vi "Convert Rectangle Data to Segment Array v2.vi"(8 "Error In":errorcluster, 9 "Box Profile Type":T1, 11 "(Rotated) Rectangle Data":i32[](array[numeric])) -> (0 "Error Out":errorcluster, 1 "Median End Points":cluster{"X":dbl, "Y":dbl}[](array[cluster]), 2 "Rectangle End Points":cluster{"X":dbl, "Y":dbl}[](array[cluster]), 3 "Rectange Profile Segments":cluster{"Segment ROI Points":i32[]}[](array[cluster]), 5 "Number of Points":i32)   [LabVIEW 2021, in "Image.lvlib"]
doc: "Converts the array of Rectangle (or Rotated Rectangle) data to an array of structures, each containing an array of (x,y) point coordinates for the corresponding \"cross-section\" segments."
uses:
  Image.lvlib
  Box Profile Type.ctl
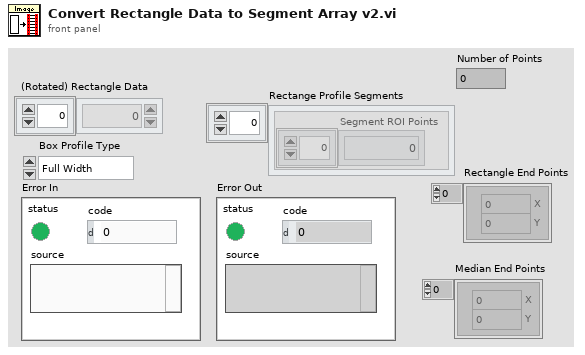
[diagram p1: front panel]
types:
  T1 = typedef "Image.lvlib/Box Profile Type.ctl" = enum16{"Full Width", "Half Width"}
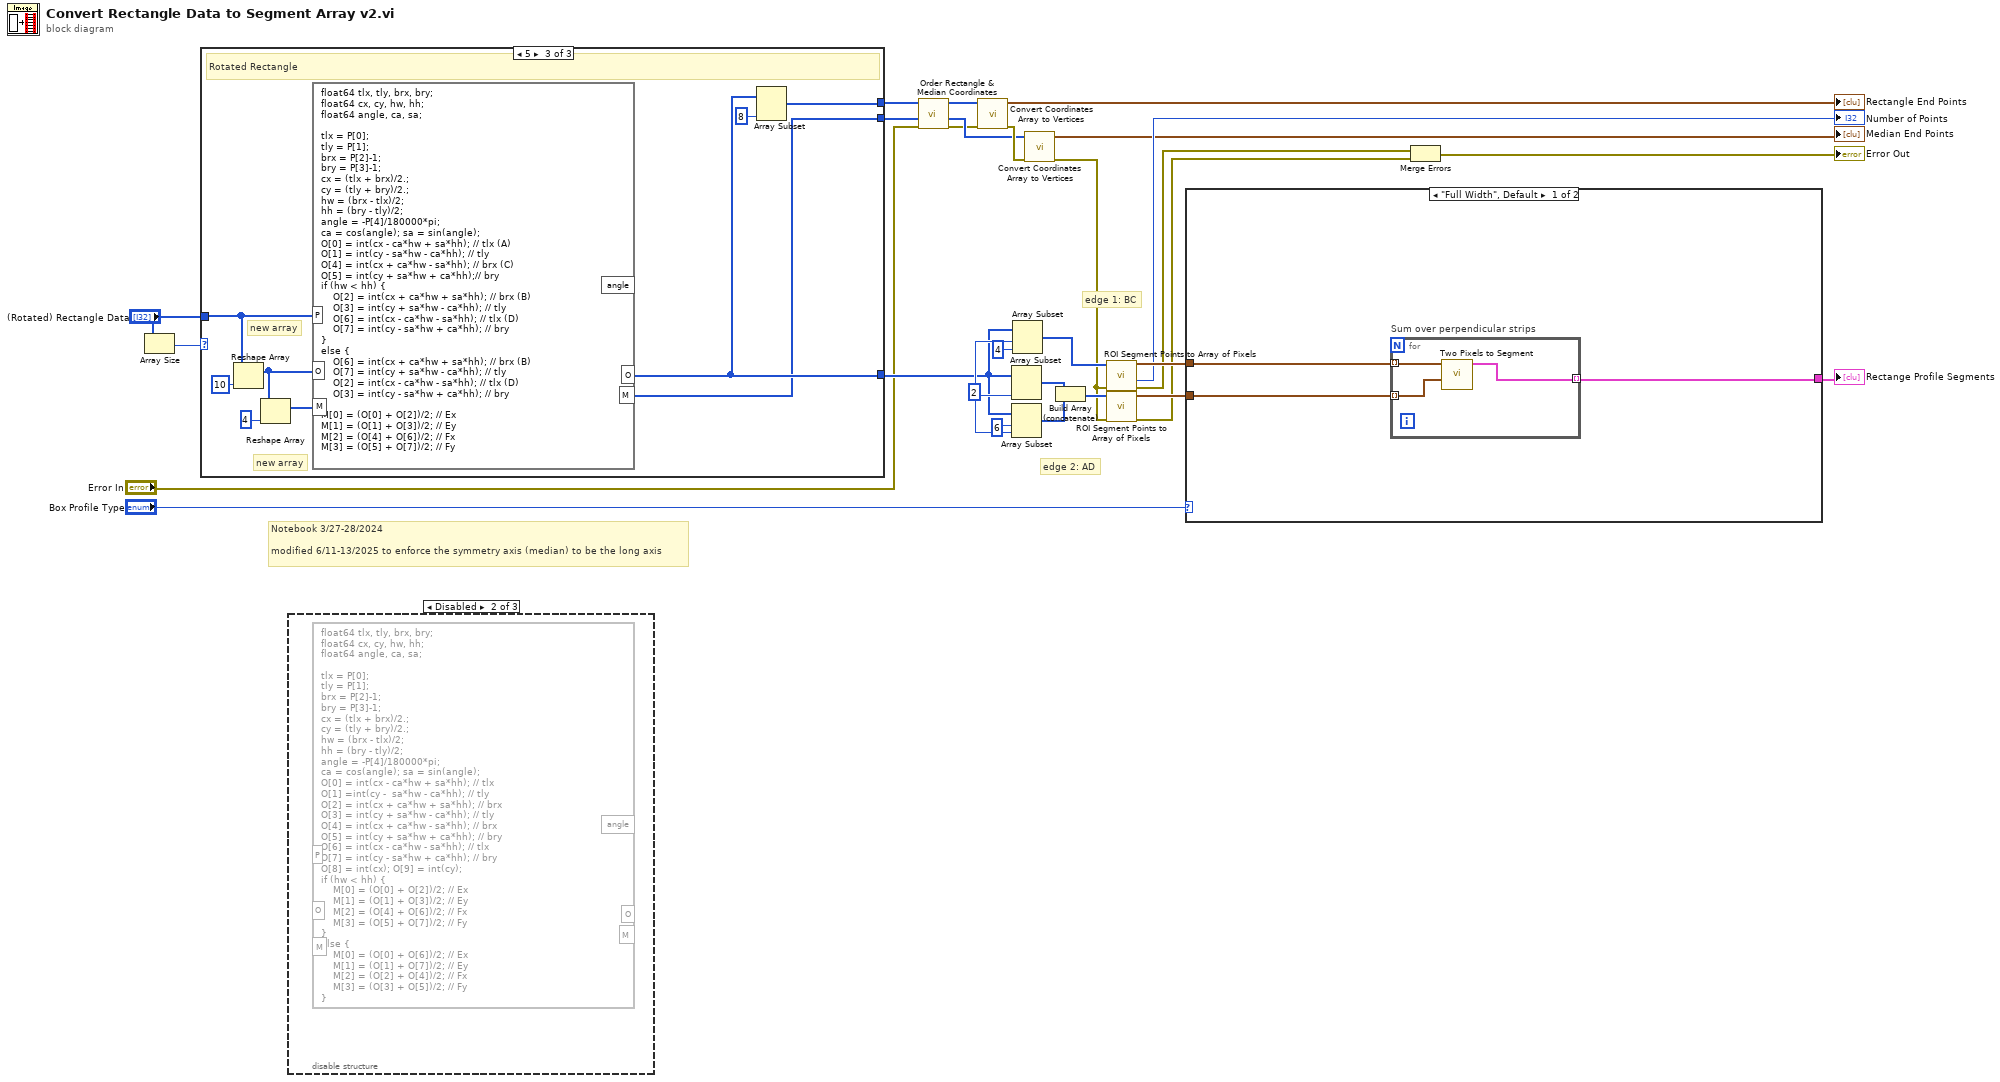
[diagram p0: block diagram]
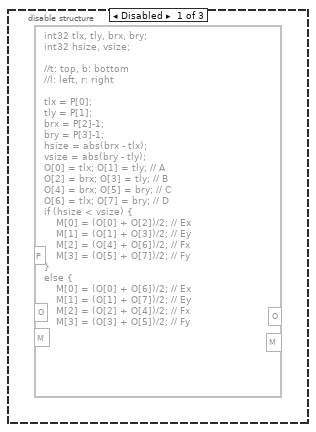
[diagram p2: hidden frame]
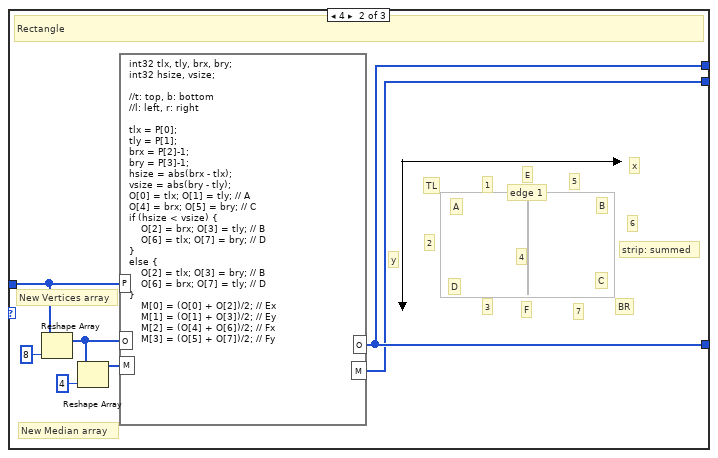
[diagram p5: hidden frame]
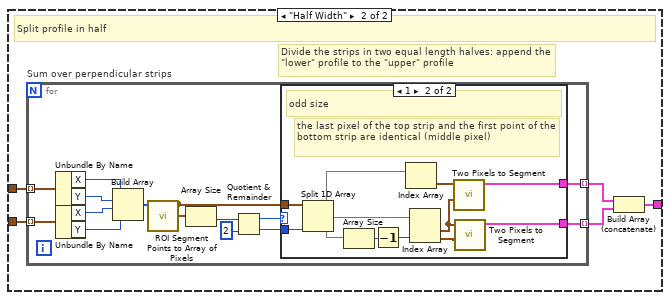
[diagram p6: hidden frame]
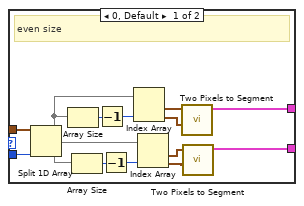
[diagram p7: hidden frame]
diagram:
  w22 = 2 ("length")
  # "edge 2: AD"
  # "edge 1: BC"
  # "Notebook 3/27-28/2024\n\nmodified 6/11-13/2025 to enforce the symmetry axis (median) to be the long axis"
  n1 = Array Size(array="(Rotated) Rectangle Data") -> (size(s)=w27:i32)
  n2 = case shown="5" w27 {
    tunnel: "(Rotated) Rectangle Data" -> [_ w35 w44]
    tunnel: [_ w33 w42] -> w12
    tunnel: [_ w33 w40] -> w6
    tunnel: [_ w29 w36] -> w5
    frame 0, Default {
    }
    frame 4 {
      # "New Median array"
      # "New Vertices array"
      # "7"
      # "6"
      # "5"
      # "4"
      # "3"
      # "2"
      # "1"
      # "F"
      # "E"
      # "strip: summed"
      # "D"
      # "C"
      # "B"
      # "A"
      # "edge 1"
      # "x"
      # "y"
      # "BR"
      # "TL"
      # "Rectangle"
      n3 = Reshape Array(w35, 8 ("dimension size")) -> (w32:i32[])
      n4 = Reshape Array(w32, 4 ("dimension size")) -> (w30:i32[])
      n5 = formula code="int32 tlx, tly, brx, bry;\nint32 hsize, vsize;\n\n//t: top, b: bottom\n//l: left, r: right\n\ntlx = P[0];\ntly = P[1];\nbrx = P[2]-1;\nbry = P[3]-1;\nhsize = abs(brx - tlx);\nvsize = abs(bry - tly);\nO[0] = tlx; O[1] = tly; // A\nO[4] = brx; O[5] = bry; // C\nif (hsize < vsize) {\n    O[2] = brx; O[3] = tly; // B\n    O[6] = tlx; O[7] = bry; // D\n}\nelse {\n    O[2] = tlx; O[3] = bry; // B\n    O[6] = brx; O[7] = tly; // D\n}\n    M[0] = (O[0] + O[2])/2; // Ex\n    M[1] = (O[1] + O[3])/2; // Ey\n    M[2] = (O[4] + O[6])/2; // Fx\n    M[3] = (O[5] + O[7])/2; // Fy"("P"=w35, "O"=w32, "M"=w30) -> ("O"=w33:i32[], "M"=w29:i32[])
    }
    frame 5 {
      # "new array"
      # "new array"
      # "Rotated Rectangle"
      n6 = Reshape Array(w44, 10 ("dimension size")) -> (w39:i32[])
      n7 = Reshape Array(w39, 4 ("dimension size")) -> (w37:i32[])
      n8 = formula code="float64 tlx, tly, brx, bry;\nfloat64 cx, cy, hw, hh;\nfloat64 angle, ca, sa;\n\ntlx = P[0];\ntly = P[1];\nbrx = P[2]-1;\nbry = P[3]-1;\ncx = (tlx + brx)/2.;\ncy = (tly + bry)/2.;\nhw = (brx - tlx)/2;\nhh = (bry - tly)/2;\nangle = -P[4]/180000*pi;\nca = cos(angle); sa = sin(angle);\nO[0] = int(cx - ca*hw + sa*hh); // tlx (A)\nO[1] = int(cy - sa*hw - ca*hh); // tly\nO[4] = int(cx + ca*hw - sa*hh); // brx (C)\nO[5] = int(cy + sa*hw + ca*hh);// bry\nif (hw < hh) {\n    O[2] = int(cx + ca*hw + sa*hh); // brx (B)\n    O[3] = int(cy + sa*hw - ca*hh); // tly\n    O[6] = int(cx - ca*hw - sa*hh); // tlx (D)\n    O[7] = int(cy - sa*hw + ca*hh); // bry\n}\nelse {\n    O[6] = int(cx + ca*hw + sa*hh); // brx (B)\n    O[7] = int(cy + sa*hw - ca*hh); // tly\n    O[2] = int(cx - ca*hw - sa*hh); // tlx (D)\n    O[3] = int(cy - sa*hw + ca*hh); // bry\n}\nM[0] = (O[0] + O[2])/2; // Ex\nM[1] = (O[1] + O[3])/2; // Ey\nM[2] = (O[4] + O[6])/2; // Fx\nM[3] = (O[5] + O[7])/2; // Fy"("P"=w44, "O"=w39, "M"=w37) -> ("O"=w42:i32[], "M"=w36:i32[])  [unwired: 1 out]
      n9 = Array Subset(array=w42, length=8) -> (w40:i32[])  [unwired: 1 in]
    }
  }
  n10 = disable-structure shown="Disabled" {
    frame Disabled {
      n11 = formula code="int32 tlx, tly, brx, bry;\nint32 hsize, vsize;\n\n//t: top, b: bottom\n//l: left, r: right\n\ntlx = P[0];\ntly = P[1];\nbrx = P[2]-1;\nbry = P[3]-1;\nhsize = abs(brx - tlx);\nvsize = abs(bry - tly);\nO[0] = tlx; O[1] = tly; // A\nO[2] = brx; O[3] = tly; // B\nO[4] = brx; O[5] = bry; // C\nO[6] = tlx; O[7] = bry; // D\nif (hsize < vsize) {\n    M[0] = (O[0] + O[2])/2; // Ex\n    M[1] = (O[1] + O[3])/2; // Ey\n    M[2] = (O[4] + O[6])/2; // Fx\n    M[3] = (O[5] + O[7])/2; // Fy\n}\nelse {\n    M[0] = (O[0] + O[6])/2; // Ex\n    M[1] = (O[1] + O[7])/2; // Ey\n    M[2] = (O[2] + O[4])/2; // Fx\n    M[3] = (O[3] + O[5])/2; // Fy\n}"() -> ()  [unwired: 3 in, 2 out]
    }
    frame Disabled {
      n12 = formula code="float64 tlx, tly, brx, bry;\nfloat64 cx, cy, hw, hh;\nfloat64 angle, ca, sa;\n\ntlx = P[0];\ntly = P[1];\nbrx = P[2]-1;\nbry = P[3]-1;\ncx = (tlx + brx)/2.;\ncy = (tly + bry)/2.;\nhw = (brx - tlx)/2;\nhh = (bry - tly)/2;\nangle = -P[4]/180000*pi;\nca = cos(angle); sa = sin(angle);\nO[0] = int(cx - ca*hw + sa*hh); // tlx\nO[1] =int(cy -  sa*hw - ca*hh); // tly\nO[2] = int(cx + ca*hw + sa*hh); // brx\nO[3] = int(cy + sa*hw - ca*hh); // tly\nO[4] = int(cx + ca*hw - sa*hh); // brx\nO[5] = int(cy + sa*hw + ca*hh); // bry\nO[6] = int(cx - ca*hw - sa*hh); // tlx\nO[7] = int(cy - sa*hw + ca*hh); // bry\nO[8] = int(cx); O[9] = int(cy);\nif (hw < hh) {\n    M[0] = (O[0] + O[2])/2; // Ex\n    M[1] = (O[1] + O[3])/2; // Ey\n    M[2] = (O[4] + O[6])/2; // Fx\n    M[3] = (O[5] + O[7])/2; // Fy\n}\nelse {\n    M[0] = (O[0] + O[6])/2; // Ex\n    M[1] = (O[1] + O[7])/2; // Ey\n    M[2] = (O[2] + O[4])/2; // Fx\n    M[3] = (O[3] + O[5])/2; // Fy\n}"() -> ()  [unwired: 3 in, 3 out]
    }
    frame Enabled {
    }
  }
  n13 = call "Order Rectangle & Median Coordinates.vi"("Error In"="Error In", "EF"=w5, "ABCD"=w6) -> ("Error Out"=w1:errorcluster, "Median"=w3:i32[], "Rectangle"=w4:i32[])  [unwired: 6 in]
  n14 = call "Convert Coordinates Array to Vertices.vi"("Error In"=w1, "Coordinates in"=w4) -> ("Error Out"=w9:errorcluster, "Vertices out"=→"Rectangle End Points":cluster{"X":dbl, "Y":dbl}[])  [unwired: 8 in]
  n15 = Array Subset(array=w12, length=w22) -> (w25:i32[])  [unwired: 1 in]
  n16 = Array Subset(array=w12, index=6, length=w22) -> (w23:i32[])
  n17 = Array Subset(array=w12, index=w22, length=4) -> (w20:i32[])
  n18 = call "Convert Coordinates Array to Vertices.vi"("Error In"=w9, "Coordinates in"=w3) -> ("Error Out"=w8:errorcluster, "Vertices out"=→"Median End Points":cluster{"X":dbl, "Y":dbl}[])  [unwired: 8 in]
  n19 = Build Array (concatenate)(w25, w23) -> (w24:i32[])
  n20 = call "ROI Segment Points to Array of Pixels.vi"("error in (no error)"=w8, "Segment ROI Points"=w20) -> ("Error Out"=w16:errorcluster, "Number of Points"=→"Number of Points":i32, "Pixels of the Segment"=w19:cluster{"X":i32, "Y":i32}[])  [unwired: 7 in]
  n21 = call "ROI Segment Points to Array of Pixels.vi"("error in (no error)"=w8, "Segment ROI Points"=w24) -> ("Error Out"=w14:errorcluster, "Pixels of the Segment"=w18:cluster{"X":i32, "Y":i32}[])  [unwired: 7 in, 1 out]
  n22 = case shown="\"Full Width\", Default" "Box Profile Type" {
    tunnel: w19 -> [w47 w54]
    tunnel: w18 -> [w46 w55]
    tunnel: [w45 w51] -> w17
    frame "Full Width", Default {
      n23 = for "Sum over perpendicular strips" {
        tunnel: w47 -> [w50] mode=indexing
        tunnel: w46 -> [w48] mode=indexing
        tunnel: [w49] -> w45 mode=indexing
        n24 = call "Two Pixels to Segment.vi"("Pixel 2"=w48, "Pixel 1"=w50) -> ("Segment 1-2"=w49:cluster{"Array":i32[]})  [unwired: 8 in, 1 out]
      }
    }
    frame "Half Width" {
      # "Divide the strips in two equal length halves: append the \"lower\" profile to the \"upper\" profile"
      # "Split profile in half"
      n25 = for "Sum over perpendicular strips" {
        tunnel: w54 -> [w69] mode=indexing
        tunnel: w55 -> [w68] mode=indexing
        tunnel: [w57] -> w53 mode=indexing
        tunnel: [w56] -> w52 mode=indexing
        n26 = Unbundle By Name(w69) -> ("X"=w67:i32, "Y"=w65:i32)
        n27 = Unbundle By Name(w68) -> ("X"=w64:i32, "Y"=w66:i32)
        n28 = Build Array(w67, w65, w64, w66) -> (w63:i32[])
        n29 = call "ROI Segment Points to Array of Pixels.vi"("Segment ROI Points"=w63) -> ("Pixels of the Segment"=w58:cluster{"X":i32, "Y":i32}[])  [unwired: 8 in, 2 out]
        n30 = Array Size(array=w58) -> (size(s)=w62:i32)
        n31 = Quotient & Remainder(x=w62, y=2) -> (x-y*floor(x/y)=w60:i32, floor(x/y)=w59:i32)
        n32 = case shown="1" w60 {
          tunnel: w59 -> [w82 w93]
          tunnel: w58 -> [w83 w94]
          tunnel: [w76 w90] -> w57
          tunnel: [w70 w85] -> w56
          frame 0, Default {
            # "even size"
            n33 = Split 1D Array(array=w83, index=w82) -> (first subarray=w81:cluster{"X":i32, "Y":i32}[], second subarray=w73:cluster{"X":i32, "Y":i32}[])
            n34 = Array Size(array=w81) -> (size(s)=w80:i32)
            n35 = Array Size(array=w73) -> (size(s)=w74:i32)
            n36 = Decrement(x=w80) -> (x-1=w79:i32)
            n37 = Decrement(x=w74) -> (x-1=w75:i32)
            n38 = Index Array(array=w81, index #2=w79) -> (element #1=w78:cluster{"X":i32, "Y":i32}, element #2=w77:cluster{"X":i32, "Y":i32})  [unwired: 1 in]
            n39 = Index Array(array=w73, index #2=w75) -> (element #1=w72:cluster{"X":i32, "Y":i32}, element #2=w71:cluster{"X":i32, "Y":i32})  [unwired: 1 in]
            n40 = call "Two Pixels to Segment.vi"("Pixel 2"=w77, "Pixel 1"=w78) -> ("Segment 1-2"=w76:cluster{"Array":i32[]})  [unwired: 8 in, 1 out]
            n41 = call "Two Pixels to Segment.vi"("Pixel 2"=w71, "Pixel 1"=w72) -> ("Segment 1-2"=w70:cluster{"Array":i32[]})  [unwired: 8 in, 1 out]
          }
          frame 1 {
            # "the last pixel of the top strip and the first point of the bottom strip are identical (middle pixel)"
            # "odd size"
            n42 = Split 1D Array(array=w94, index=w93) -> (first subarray=w92:cluster{"X":i32, "Y":i32}[], second subarray=w87:cluster{"X":i32, "Y":i32}[])
            n43 = Array Size(array=w87) -> (size(s)=w88:i32)
            n44 = Decrement(x=w88) -> (x-1=w89:i32)
            n45 = Index Array(array=w92) -> (element=w91:cluster{"X":i32, "Y":i32})  [unwired: 1 in]
            n46 = Index Array(array=w87, index #2=w89) -> (element #1=w84:cluster{"X":i32, "Y":i32}, element #2=w86:cluster{"X":i32, "Y":i32})  [unwired: 1 in]
            n47 = call "Two Pixels to Segment.vi"("Pixel 2"=w84, "Pixel 1"=w91) -> ("Segment 1-2"=w90:cluster{"Array":i32[]})  [unwired: 8 in, 1 out]
            n48 = call "Two Pixels to Segment.vi"("Pixel 2"=w86, "Pixel 1"=w84) -> ("Segment 1-2"=w85:cluster{"Array":i32[]})  [unwired: 8 in, 1 out]
          }
        }
      }
      n49 = Build Array (concatenate)(w53, w52) -> (w51:cluster{"Array":i32[]}[])
    }
  }
  "Rectange Profile Segments" <- w17
  n50 = Merge Errors(w16, w14) -> (→"Error Out":errorcluster)
